vi "getGlyphFile.vi"(8 "error in (no error)":errorcluster, 11 "Category in":refnum<class "Category.lvclass">) -> (0 "error out":errorcluster, 2 "Glyph File":string, 3 "Category out":refnum<class "Category.lvclass">)   [LabVIEW 2013, in "Category.lvclass"]
doc: "Dynamic Dispatch VI. Returns the name of the glyph file to be used as a glyph in the tree control. A empty string means no glyph."
uses:
  Category.lvclass
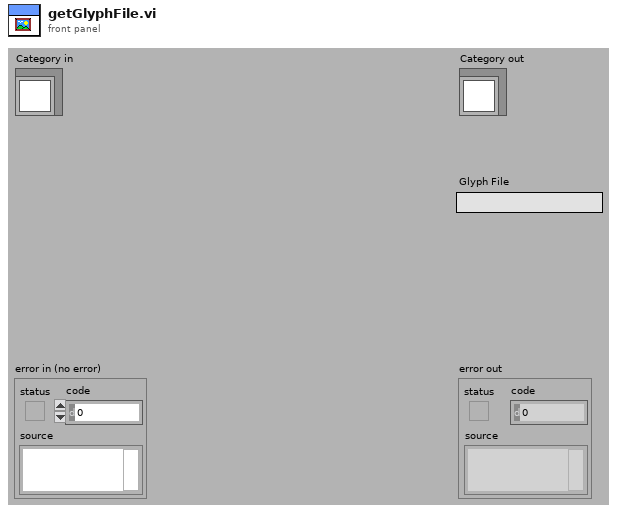
[diagram p1: front panel]
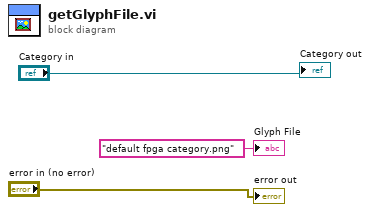
[diagram p0: block diagram]
diagram:
  "error out" <- "error in (no error)"
  "Category out" <- "Category in"
  "Glyph File" <- "default fpga category.png" ("Glyph File")
